vi "Read Element of PID per ID.vi"(8 "error in (no error)":errorcluster, 10 "index":i32, 11 "Parameters in":refnum<class "Parameters.lvclass">) -> (0 "error out":errorcluster, 2 "PID Parameters":T1={"PID gains Vel D"={"(Kp)"=0.4, "(Ki)"=1e-06, "(Kd)"=0.65}, "PID gains Angle"={"(Kc)"=4.5, "(Ki)"=0.0, "(Kd)"=0.0001}, "PID gains Angle To Turn"={"(Kc)"=4.0, "(Ki)"=1e-05, "(Kd)"=0.012}, "PID gains Lateral"={"(Kc)"=2.0, "(Ki)"=0.0, "(Kd)"=0.001}}, 3 "Parameters out":refnum<class "Parameters.lvclass">)   [LabVIEW 2024, in "Parameters.lvclass"]
uses:
  Parameters.lvclass
  Controls/PIDParameters.ctl
  Parameters.lvclass/Parameters.ctl
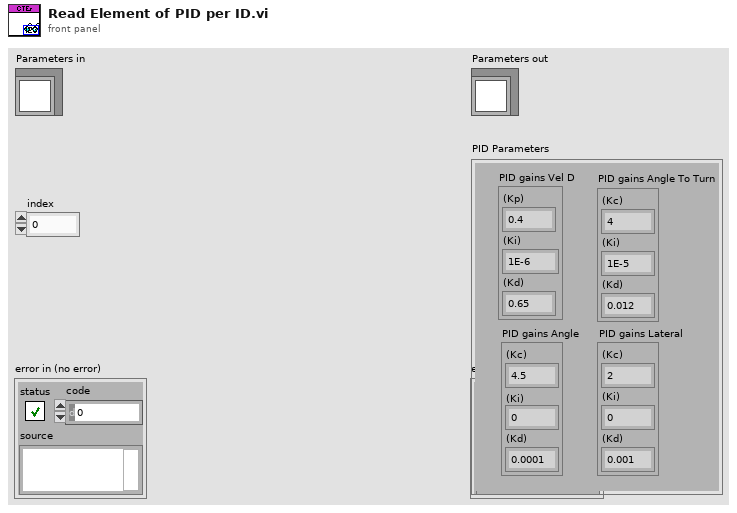
[diagram p1: front panel]
types:
  T1 = typedef "PIDParameters.ctl" = cluster{"PID gains Vel D":cluster{"(Kp)":dbl, "(Ki)":dbl, "(Kd)":dbl}, "PID gains Angle":cluster{"(Kc)":dbl, "(Ki)":dbl, "(Kd)":dbl}, "PID gains Angle To Turn":cluster{"(Kc)":dbl, "(Ki)":dbl, "(Kd)":dbl}, "PID gains Lateral":cluster{"(Kc)":dbl, "(Ki)":dbl, "(Kd)":dbl}}
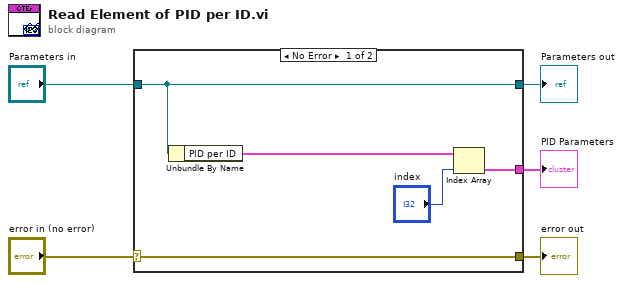
[diagram p0: block diagram]
diagram:
  n1 = case shown="No Error" "error in (no error)" {
    selector: "error in (no error)" -> [w10 w11]
    tunnel: [w10 w11] -> w4
    tunnel: [w9 w12] -> w2
    tunnel: "Parameters in" -> [w9 w12]
    tunnel: [w6 _] -> w1
    frame No Error {
      n2 = Unbundle By Name(w9) -> ("PID per ID"=w8:T1[])
      n3 = Index Array(array=w8, index="index") -> (element=w6:T1)
    }
    frame Error {
    }
  }
  "error out" <- w4
  "Parameters out" <- w2
  "PID Parameters" <- w1
